vi "Test_conditioning_circuitvi.vi"() -> ()   [LabVIEW 2021]
uses:
  <vilib>/Platform/TimedLoop/XDataNode/timing_clust.ctl
  <vilib>/Platform/TimedLoop/XDataNode/nitl_modes.ctl
  <vilib>/Platform/TimedLoop/XDataNode/wakeup.ctl
  <vilib>/myRIO/Instrument Drivers/Onboard IO/AO/typedefs/AO Reference.ctl
  <vilib>/myRIO/Common/Instrument Driver Framework/Utilities/typedefs/myRIO Generic Hardware Reference.ctl
  <vilib>/myRIO/Common/Instrument Driver Framework/Utilities/typedefs/Hardware Version Enum.ctl
  <vilib>/myRIO/Common/Instrument Driver Framework/Utilities/typedefs/myRIO v1.0 Reference.ctl
  <vilib>/myRIO/Common/Instrument Driver Framework/Utilities/typedefs/Generic FPGA Reference.ctl
  <vilib>/myRIO/Common/Instrument Driver Framework/myRIO v1.0/AO/typedefs/AO Channels List.ctl
  <vilib>/myRIO/Common/Instrument Driver Framework/myRIO v1.0/AO/typedefs/AO Channels Enum.ctl
  <vilib>/myRIO/Common/Instrument Driver Framework/Utilities/typedefs/Analog Scaling Constants List.ctl
  <vilib>/myRIO/Common/Instrument Driver Framework/Utilities/typedefs/Analog Scaling Constants.ctl
  <vilib>/userDefined/High Color/nirio_resource_hc.ctl
  <vilib>/myRIO/Instrument Drivers/Onboard IO/AI/typedefs/AI Reference.ctl
  <vilib>/myRIO/Common/Instrument Driver Framework/myRIO v1.0/AI/typedefs/AI Channels List.ctl
  <vilib>/myRIO/Common/Instrument Driver Framework/myRIO v1.0/AI/typedefs/AI Channels Enum.ctl
  <vilib>/myRIO/Common/Instrument Driver Framework/Utilities/vis/Is FPGA Ref Available.vi
  <vilib>/myRIO/Common/Instrument Driver Framework/myRIO v1.0/AO/vis/myRIO v1.1 Open AO.vi
  <vilib>/myRIO/Instrument Drivers/Onboard IO/AO/vis/Write.vi
  <vilib>/myRIO/Common/Instrument Driver Framework/myRIO v1.0/AI/vis/myRIO v1.1 Open AI.vi
  <vilib>/myRIO/Instrument Drivers/Onboard IO/AI/vis/Read.vi
  <vilib>/myRIO/Common/Instrument Driver Framework/Utilities/vis/Validate Channels.vi
  <vilib>/myRIO/Common/Instrument Driver Framework/myRIO v1.0/AO/vis/myRIO v1.0 Reserve AO.vi
  <vilib>/myRIO/Common/Instrument Driver Framework/myRIO v1.0/AI/vis/myRIO v1.0 Reserve AI.vi
  <vilib>/myRIO/Common/Instrument Driver Framework/myRIO v1.0/AO/vis/myRIO v1.0 Build MUX Configuration AO.vi
  <vilib>/myRIO/Common/Instrument Driver Framework/myRIO v1.0/Resource Manager/vis/myRIO v1.0 Reserve Channel List.vi
  <vilib>/myRIO/Common/Instrument Driver Framework/myRIO v1.0/AI/vis/myRIO v1.0 Build MUX Configuration AI.vi
  <vilib>/myRIO/Common/Instrument Driver Framework/myRIO v1.0/Resource Manager/vis/myRIO v1.0 Reserve Channel.vi
  <vilib>/myRIO/Common/Instrument Driver Framework/myRIO v1.0/Resource Manager/vis/myRIO v1.0 Unreserve Channel.vi
  <vilib>/myRIO/Common/Instrument Driver Framework/myRIO v1.0/Resource Manager/vis/myRIO v1.0 Build Mutex Name.vi
  <vilib>/Utility/VariantDataType/GetNumericInfo.vi
  <vilib>/Utility/error.llb/Error Cluster From Error Code.vi
  <vilib>/myRIO/Common/Instrument Driver Framework/myRIO v1.0/myRIO v1.1 Open.vi
  <vilib>/myRIO/Common/Instrument Driver Framework/myRIO v1.0/AO/vis/myRIO v1.0 Get Scaling Constants AO.vi
  <vilib>/myRIO/Common/Instrument Driver Framework/Utilities/vis/IO Manager.vi
  <vilib>/myRIO/Common/Instrument Driver Framework/Utilities/vis/Configuration Manager.vi
  <vilib>/myRIO/Common/Instrument Driver Framework/myRIO v1.0/myRIO v1.0 Close.vi
  <vilib>/myRIO/Common/Instrument Driver Framework/myRIO v1.0/AO/vis/myRIO v1.0 Write AO.vi
  <vilib>/myRIO/Common/Instrument Driver Framework/myRIO v1.0/AI/vis/myRIO v1.0 Get Scaling Constants AI.vi
  <vilib>/myRIO/Common/Instrument Driver Framework/myRIO v1.0/AI/vis/myRIO v1.0 Read AI.vi
  <vilib>/Platform/TimedLoop/XDataNode/XDataNode.xnode
  <vilib>/myRIO/Express VI/Onboard IO/AO/AO Express VI.xnode
  <vilib>/myRIO/Instrument Drivers/Onboard IO/AO/vis/myRIO AO Open.xnode
  <vilib>/myRIO/Express VI/Onboard IO/AI/AI Express VI.xnode
  <vilib>/myRIO/Instrument Drivers/Onboard IO/AI/vis/myRIO AI Open.xnode
  <vilib>/Analysis/NI_AALBase.lvlib
  <vilib>/myRIO/Instrument Drivers/Onboard IO/AO/AO.lvlib
  <vilib>/Platform/TimedLoop/XDataNode/XDNodeRunTimeDep.lvlib
  <vilib>/myRIO/Instrument Drivers/Onboard IO/AI/AI.lvlib
panel:
  in  "Tab Control":enum32{"Fgen Test", "Signal Conditioning Test"}(tab)
  in  "dt (ms)":i64
  in  "Frequency 2":dbl=1.0 format="%0.2f"
  in  "Amplitude 2":dbl=1.0 format="%0.2f"
  out "Analog Output Signal 2":dbl(graph)
  out "Ofset Fgen Waveform":dbl[](graph)
  in  "stop 2":bool
  out "Current Value 2":dbl
  out "# cycles":dbl
  in  "Offset 2":dbl=1.0 format="%0.2f"
  out "Test Vpp":dbl
  out "Original Fgen Waveform":dbl[](graph)
  out "R Vpp":dbl
  out "R Channel (Pin 3)":dbl(graph)
  out "Analog Output Waveform":dbl(graph)
  out "Fgen Waveform":dbl[](graph)
  in  "stop":bool
  in  "Amplitude":dbl=1.0 format="%0.2f"
  in  "Frequency":dbl=1.0 format="%0.2f"
  in  "# Sample / Cycle":i32=128
  in  "# Cycle":dbl=100.0
  out "Current Fgen Value":dbl
  out "IR Channel (Pin 5)":dbl(graph)
  in  "Offset":dbl=1.0 format="%0.2f"
  out "IR Vpp":dbl
  out "dt":dbl
  # "Default # Sample: 128"
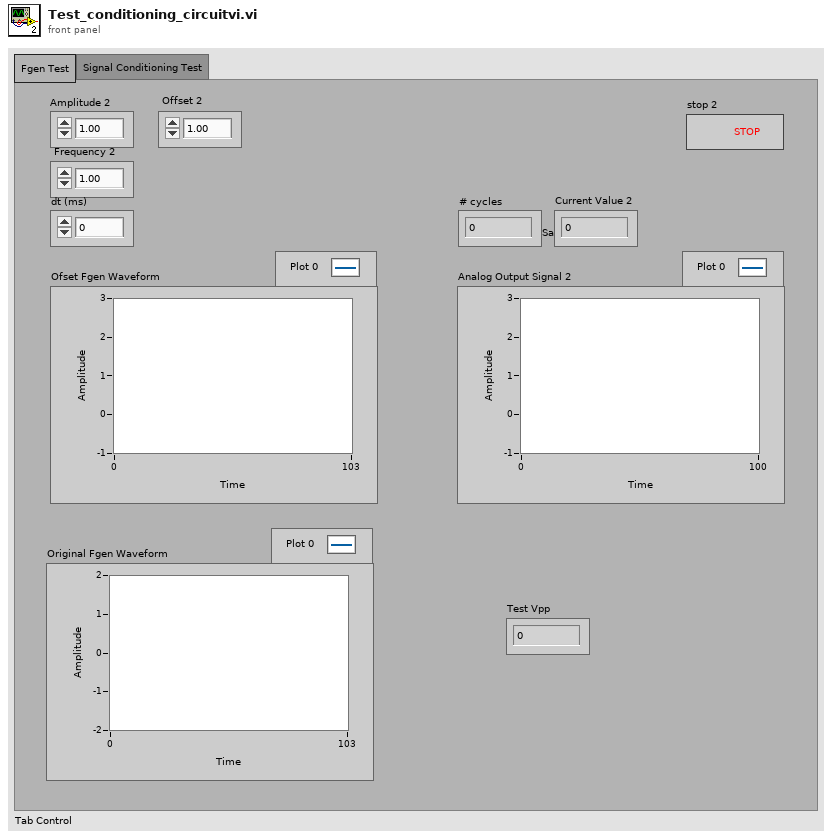
[diagram p1: front panel]
types:
  T1 = typedef "XDNodeRunTimeDep.lvlib/timing_clust.ctl" = cluster{"Expected End [f-1]":u64, "Actual End [f-1]":u64, "Finished Late? [f-1]":bool, "Expected End [i-1]":u64, "Actual End [i-1]":u64, "Finished Late? [i-1]":bool, "Expected Start [i]":u64, "Actual Start [i]":u64, "Expected Start [f]":u64, "Actual Start [f]":u64, "Source Name":string, "Structure Name":string, "Period":i64, "Deadline":i64, "Offset":i64, "Start":i64, "Priority":i32, "Timeout":i32, "Mode":T2, "Wakeup Reason":T3, "Error":errorcluster, "Source Type":string, "Secondary Source Type":string, "Global End Time":u64, "Global Start Time":u64, "Frame Duration":u64, "Iteration Duration":u64, "Assigned CPU":i32, "I/O Scan Engine Mode":u32}
  T2 = typedef "XDNodeRunTimeDep.lvlib/nitl_modes.ctl" = enum32{"No Change", "Process missed periods, maintain original phase", "Discard missed periods, maintain original phase", "Process missed periods, ignore original phase", "Discard missed periods, ignore original phase"}
  T3 = typedef "XDNodeRunTimeDep.lvlib/wakeup.ctl" = enum32{"Normal", "Aborted", "Asynchronous wakeup", "Timing source error", "Timed loop error", "Timeout"}
  T4 = typedef "AO.lvlib/AO Reference.ctl" = cluster{"myRIO Reference":T5, "AO Channel List":T9, "AO Scaling Constant List":T11}
  T5 = typedef "myRIO Generic Hardware Reference.ctl" = cluster{"myRIO Model":T6, "myRIO Hardware Reference":T7}
  T6 = typedef "Hardware Version Enum.ctl" = enum16{"Unknown", "myRIO-1900", "myRIO-1950", "roboRIO", "NI ELVIS RIO CM", "ELVIS III"}
  T7 = typedef "myRIO v1.0 Reference.ctl" = cluster{"Generic FPGA Reference":T8, "Allow multiple opens":bool}
  T8 = typedef "Generic FPGA Reference.ctl" = refnum<k20>
  T9 = typedef "AO Channels List.ctl" = T10[]
  T10 = typedef "AO Channels Enum.ctl" = enum16{"Not Connected", "AudioOut/Left", "AudioOut/Right", "C/AO0", "C/AO1", "A/AO0", "A/AO1", "B/AO0", "B/AO1"}
  T11 = typedef "Analog Scaling Constants List.ctl" = T12[]
  T12 = typedef "Analog Scaling Constants.ctl" = cluster{"LSB Weight (Volts)":dbl, "Offset (Volts)":dbl, "Signed?":bool}
  T13 = typedef "nirio_resource_hc.ctl" = tag
  T14 = typedef "AI.lvlib/AI Reference.ctl" = cluster{"myRIO Reference":T5, "AI Channels List":T15, "AI Scaling Constants List":T11}
  T15 = typedef "AI Channels List.ctl" = T16[]
  T16 = typedef "AI Channels Enum.ctl" = enum16{"Not Connected", "AudioIn/Left", "AudioIn/Right", "C/AI0", "C/AI1", "A/AI0", "A/AI1", "A/AI2", "A/AI3", "A/AI4", "A/AI5", "A/AI6", "A/AI7", "B/AI0", "B/AI1", "B/AI2", "B/AI3", "B/AI4", "B/AI5", "B/AI6", "B/AI7", "AI/AI0", "AI/AI1", "AI/AI2", "AI/AI3", "A/AI0 (DIFF)", "A/AI1 (DIFF)", "A/AI2 (DIFF)", "A/AI3 (DIFF)", "B/AI0 (DIFF)", "B/AI1 (DIFF)", "B/AI2 (DIFF)", "B/AI3 (DIFF)"}
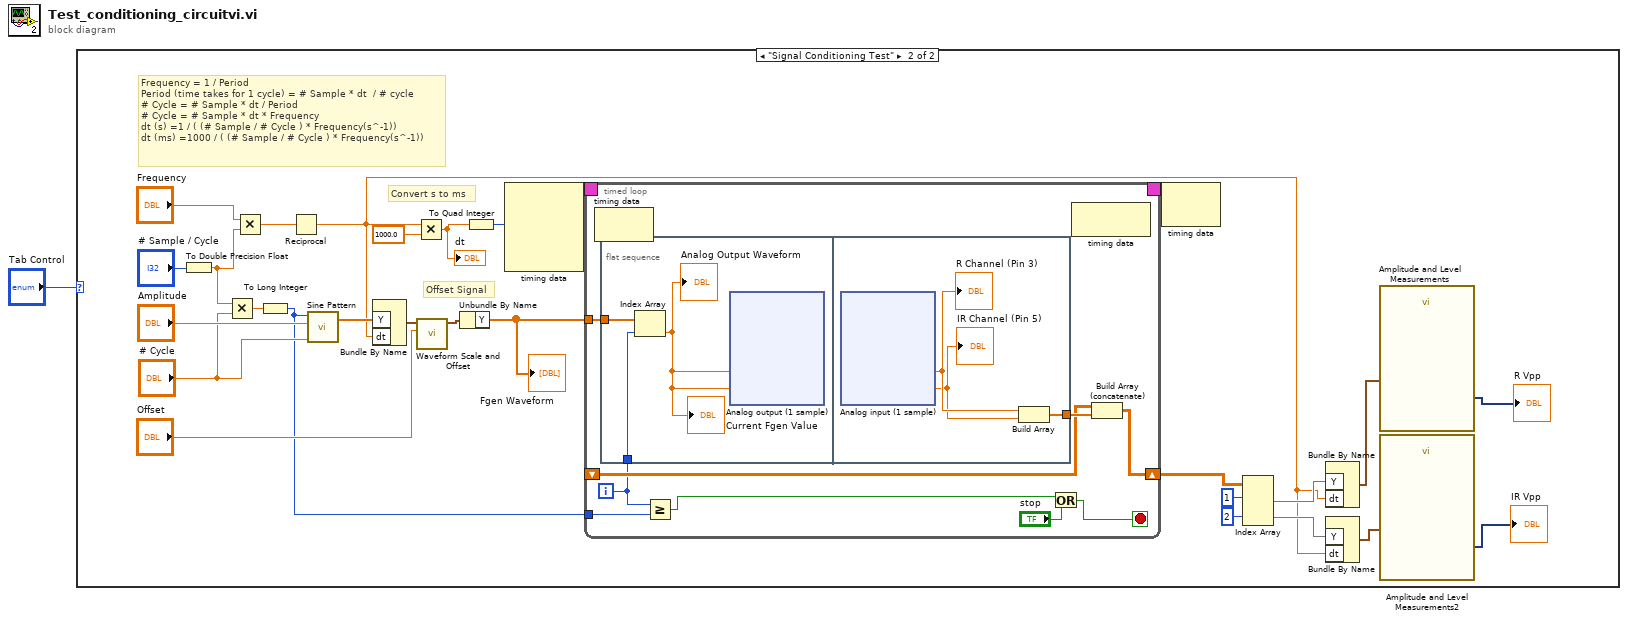
[diagram p0: block diagram]
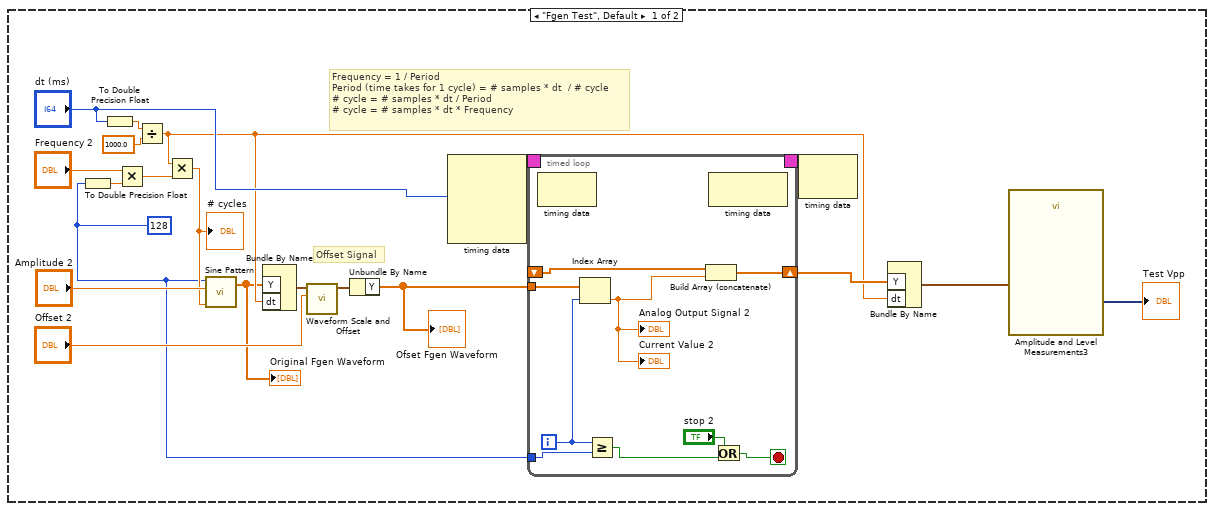
[diagram p2: hidden frame]
diagram:
  n1 = case shown="\"Signal Conditioning Test\"" "Tab Control" {
    frame "Fgen Test", Default {
      w3 = 128 ("samples")
      # "Offset Signal"
      # "Frequency = 1 / Period\nPeriod (time takes for 1 cycle) = # samples * dt  / # cycle\n# cycle = # samples * dt / Period\n# cycle = # samples * dt * Frequency"
      n2 = To Double Precision Float(number=w3) -> (double precision float=w17:dbl)
      n3 = To Double Precision Float(number="dt (ms)") -> (double precision float=w13:dbl)
      n4 = Multiply(x="Frequency 2", y=w17) -> (x*y=w16:dbl)
      n5 = Divide(x=w13, y=1000.0) -> (x/y=w6:dbl)
      n6 = Multiply(x=w6, y=w16) -> (x*y=w8:dbl)
      "# cycles" <- w8
      n7 = call <vilib>:"Sine Pattern.vi"("cycles"=w8, "amplitude"="Amplitude 2", "samples"=w3) -> ("Sinusoidal Pattern"=w2:dbl[])  [unwired: 1 in, 1 out]
      "Original Fgen Waveform" <- w2
      n8 = Bundle By Name("Y"=w2, "dt"=w6) -> (w12:waveform(dbl))  [unwired: 1 in]
      n9 = call <vilib>:"Waveform Scale and Offset.vi"("offset"="Offset 2", "waveform in"=w12) -> ("waveform out"=w10:waveform(dbl))  [unwired: 8 in, 1 out]
      n10 = Unbundle By Name(w10) -> ("Y"=w9:dbl[])
      "Ofset Fgen Waveform" <- w9
      n11 = node-c288("dt (ms)") -> (w21:T1)  [unwired: 3 in]
      n12 = timed-loop {
        timing: w21 -> [_]
        timing-out: [_] -> w20
        tunnel: w9 -> [w30]
        shift-right: [w28] -> w7
        shift-left: _ -> [w27]
        tunnel: w3 -> [w25]
        i -> [w26]
        stop <- w22 stop-if-true
        n13 = node-c288() -> ()  [unwired: 1 in, 1 out]
        n14 = Index Array(array=w30, index=w26) -> (element=w29:dbl)
        "Analog Output Signal 2" <- w29
        "Current Value 2" <- w29
        n15 = Greater Or Equal?(x=w26, y=w25) -> (x >= y?=w23:bool)
        n16 = Build Array (concatenate)(w27, w29) -> (w28:dbl[])
        n17 = node-c288() -> ()  [unwired: 1 in, 1 out]
        n18 = Or(x="stop 2", y=w23) -> (x .or. y?=w22:bool)
      }
      n19 = node-c288(w20) -> ()  [unwired: 1 out]
      n20 = Bundle By Name("Y"=w7, "dt"=w6) -> (w4:waveform(dbl))  [unwired: 1 in]
      n21 = call "Amplitude and Level Measurements3"("Signals"=w4) -> ("Peak to Peak"=→"Test Vpp":dynamicdata)  [unwired: 12 in, 2 out]
    }
    frame "Signal Conditioning Test" {
      # "Convert s to ms"
      # "Offset Signal"
      # "Frequency = 1 / Period\nPeriod (time takes for 1 cycle) = # Sample * dt  / # cycle\n# Cycle = # Sample * dt / Period\n# Cycle = # Sample * dt * Frequency\ndt (s) =1 / ( (# Sample / # Cycle ) * Frequency(s^-1))\ndt (ms) =1000 / ( (# Sample / # Cycle ) * Frequency(s^-1))"
      n22 = To Double Precision Float(number="# Sample / Cycle") -> (double precision float=w58:dbl)
      n23 = Multiply(x=w58, y="# Cycle") -> (x*y=w60:dbl)
      n24 = Multiply(x="Frequency", y=w58) -> (x*y=w50:dbl)
      n25 = To Long Integer(number=w60) -> (32bit integer=w41:i32)
      n26 = Reciprocal(x=w50) -> (1/x=w42:dbl)
      n27 = call <vilib>:"Sine Pattern.vi"("cycles"="# Cycle", "amplitude"="Amplitude", "samples"=w41) -> ("Sinusoidal Pattern"=w48:dbl[])  [unwired: 1 in, 1 out]
      n28 = Bundle By Name("Y"=w48, "dt"=w42) -> (w49:waveform(dbl))  [unwired: 1 in]
      n29 = Multiply(x=w42, y=1000.0) -> (x*y=w44:dbl)
      "dt" <- w44
      n30 = call <vilib>:"Waveform Scale and Offset.vi"("offset"="Offset", "waveform in"=w49) -> ("waveform out"=w46:waveform(dbl))  [unwired: 8 in, 1 out]
      n31 = Unbundle By Name(w46) -> ("Y"=w45:dbl[])
      "Fgen Waveform" <- w45
      n32 = To Quad Integer(1:w44) -> (0:w57:i64)
      n33 = node-c288(w57) -> (w64:T1)  [unwired: 3 in]
      n34 = timed-loop {
        timing: w64 -> [_]
        timing-out: [_] -> w63
        tunnel: w45 -> [w73]
        shift-right: [w70] -> w55
        shift-left: _ -> [w71]
        tunnel: w41 -> [w68]
        i -> [w69]
        stop <- w65 stop-if-true
        n35 = node-c288() -> ()  [unwired: 1 in, 1 out]
        n36 = flat-sequence {
          tunnel: w69 -> [w76]
          tunnel: w73 -> [w75]
          tunnel: [w115] -> w72
          frame #0 {
            n37 = Index Array(array=w75, index=w76) -> (element=w74:dbl)
            "Analog Output Waveform" <- w74
            "Current Fgen Value" <- w74
            n38 = xnode "Analog output (1 sample)"("A/AO0 (Pin 2)"=w74, "A/AO1 (Pin 4)"=w74) -> ()  [unwired: 1 in, 1 out]
          }
          frame #1 {
            n39 = xnode "Analog input (1 sample)"() -> ("A/AI0 (Pin 3)"=w117:dbl, "A/AI1 (Pin 5)"=w116:dbl)  [unwired: 1 in, 1 out]
            "R Channel (Pin 3)" <- w117
            "IR Channel (Pin 5)" <- w116
            n40 = Build Array(w117, w116) -> (w115:dbl[])
          }
        }
        n41 = Greater Or Equal?(x=w69, y=w68) -> (x >= y?=w66:bool)
        n42 = Or(x=w66, y="stop") -> (x .or. y?=w65:bool)
        n43 = node-c288() -> ()  [unwired: 1 in, 1 out]
        n44 = Build Array (concatenate)(w71, w72) -> (w70:dbl[][])
      }
      n45 = node-c288(w63) -> ()  [unwired: 1 out]
      n46 = Index Array(array=w55, index (row) #1=1 ("index (row)"), index (row) #2=2 ("index (row)")) -> (element #1=w52:dbl[], element #2=w51:dbl[])  [unwired: 2 in]
      n47 = Bundle By Name("Y"=w52, "dt"=w42) -> (w40:waveform(dbl))  [unwired: 1 in]
      n48 = Bundle By Name("Y"=w51, "dt"=w42) -> (w39:waveform(dbl))  [unwired: 1 in]
      n49 = call "Amplitude and Level Measurements"("Signals"=w40) -> ("Peak to Peak"=→"R Vpp":dynamicdata)  [unwired: 12 in, 2 out]
      n50 = call "Amplitude and Level Measurements2"("Signals"=w39) -> ("Peak to Peak"=→"IR Vpp":dynamicdata)  [unwired: 12 in, 2 out]
    }
  }
